vi "Delta_heading_wrapper.vi"(8 "Goal Heading":dbl(knob) scale=180.0..-179.0, 11 "Robot Heading":dbl(knob) scale=180.0..-179.0) -> (1 "Heading Adjustment":dbl(knob) scale=180.0..-179.0)   [LabVIEW 2012]
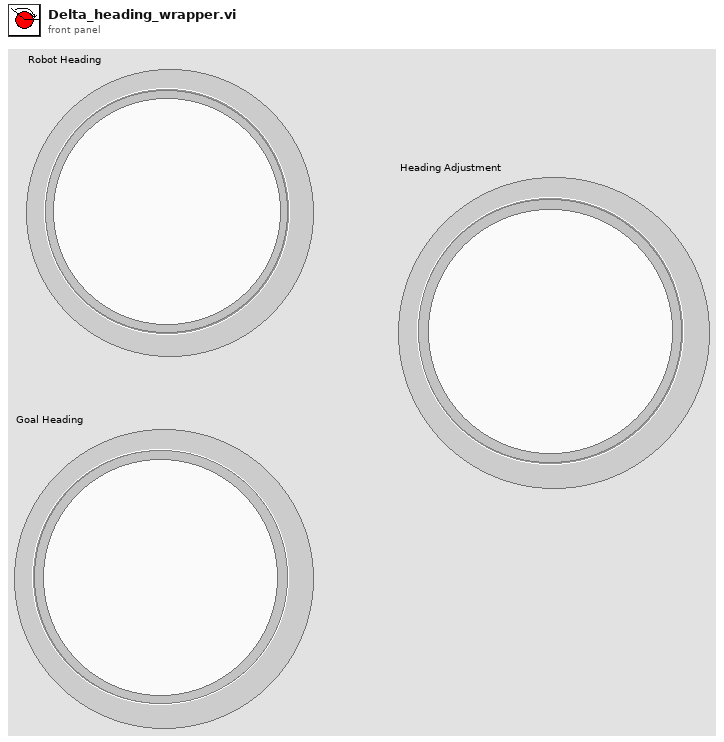
[diagram p1: front panel]
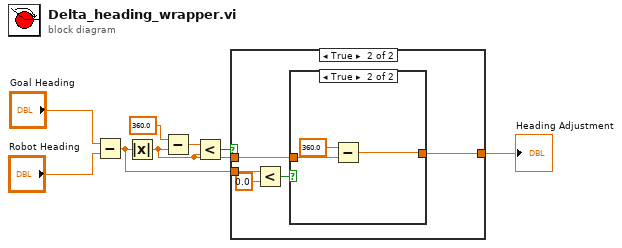
[diagram p0: block diagram]
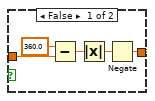
[diagram p3: hidden frame]
diagram:
  n1 = Subtract(x="Goal Heading", y="Robot Heading") -> (x-y=w5:dbl)
  n2 = Absolute Value(x=w5) -> (abs(x)=w1:dbl)
  n3 = Subtract(x=360.0, y=w1) -> (x-y=w7:dbl)
  n4 = Less?(x=w7, y=w1) -> (x < y?=w6:bool)
  n5 = case shown="True" w6 {
    tunnel: w5 -> [w9 w12]
    tunnel: [w9 w10] -> w4
    tunnel: w1 -> [_ w11]
    frame False {
    }
    frame True {
      n6 = Less?(x=w12, y=0.0) -> (x < y?=w13:bool)
      n7 = case shown="True" w13 {
        tunnel: w11 -> [w18 w21]
        tunnel: [w15 w20] -> w10
        frame False {
          n8 = Subtract(x=360.0, y=w18) -> (x-y=w17:dbl)
          n9 = Absolute Value(x=w17) -> (abs(x)=w16:dbl)
          n10 = Negate(x=w16) -> (-x=w15:dbl)
        }
        frame True {
          n11 = Subtract(x=360.0, y=w21) -> (x-y=w20:dbl)
        }
      }
    }
  }
  "Heading Adjustment" <- w4
